vi "Zoom.vi"(2 "Final Zoom":sgl, 3 "Scene.Object IN":refnum<vi>) -> (1 "Scene.Object Out":refnum<vi>)   [LabVIEW 2010]
uses:
  <vilib>/Utility/miscctls.llb/LV3DPointTypeDef.ctl
  LVPresent_Globals.vi
  <vilib>/picture/3D Picture Control/NI_3D Picture Control.lvlib
panel:
  out "Transformation:Get Scale 2":T1
  out "Array":T1[](array[typedef])
  out "Transformation:Get Scale":T1
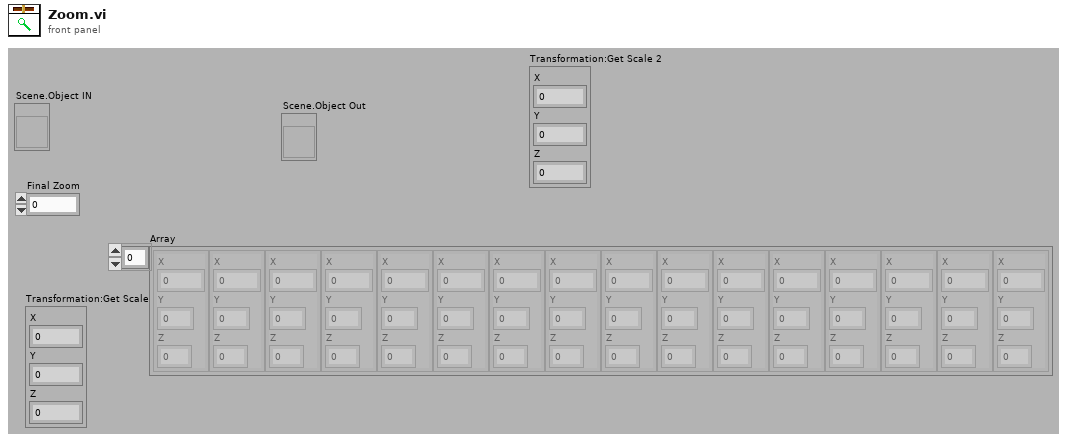
[diagram p1: front panel]
types:
  T1 = typedef "LV3DPointTypeDef.ctl" = cluster{"X":sgl, "Y":sgl, "Z":sgl}
  T2 = cluster{"Final Zoom":sgl, "Final Zoom":sgl, "Final Zoom":sgl}
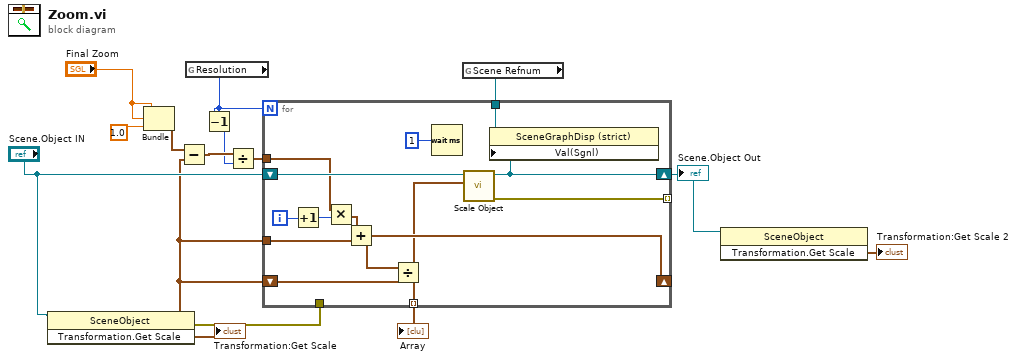
[diagram p0: block diagram]
diagram:
  n1 = invoke class="SceneObject" method="Transformation.Get Scale"(reference="Scene.Object IN") -> (error out=w6:errorcluster, "Transformation.Get Scale"=w8:T1)  [unwired: 2 in, 1 out]
  "Transformation:Get Scale" <- w8
  n2 = Bundle("Final Zoom"="Final Zoom", "Final Zoom"="Final Zoom", "Final Zoom"=sgl 1.0) -> (w13:T2)  [unwired: 1 in]
  n3 = Subtract(x=w13, y=w8) -> (x-y=w14:T1)
  n4 = global read "LVPresent_Globals.vi" "Resolution"() -> (w2:i32)
  n5 = Decrement(x=w2) -> (x-1=w1:i32)
  n6 = Divide(x=w14, y=w1) -> (x/y=w9:T1)
  n7 = global read "LVPresent_Globals.vi" "Scene Refnum"() -> (w3:refnum<vi>)
  n8 = for {
    N: w2 -> [_]
    shift-right: [w24] -> w5
    shift-left: "Scene.Object IN" -> [w20]
    tunnel: w8 -> [w25]
    tunnel: w3 -> [w23]
    shift-right: [w17] -> _
    shift-left: w8 -> [w18]
    tunnel: w9 -> [w19]
    tunnel: [w16] -> w7 mode=indexing
    tunnel: [w15] -> _ mode=indexing
    tunnel: w6 -> [_]
    i -> [w27]
    n9 = Increment(x=w27) -> (x+1=w26:i32)
    n10 = Multiply(x=w19, y=w26) -> (x*y=w21:T1)
    n11 = Add(x=w21, y=w25) -> (x+y=w17:T1)
    n12 = Divide(x=w17, y=w18) -> (x/y=w16:T1)
    n13 = Wait (ms)(milliseconds to wait=u32 1) -> ()  [unwired: 1 out]
    n14 = call <vilib>:"Scale Object.vi"("Scale"=w16, "Scene.Object In"=w20) -> ("error out"=w15:errorcluster, "Scene.Object Out"=w24:refnum<vi>)  [unwired: 8 in]
    n15 = property class="SceneGraphDisp (strict)"(reference=w23, "Val(Sgnl)"=w24) -> ()  [unwired: 1 in, 2 out]
  }
  "Scene.Object Out" <- w5
  "Array" <- w7
  n16 = invoke class="SceneObject" method="Transformation.Get Scale"(reference=w5) -> ("Transformation.Get Scale"=→"Transformation:Get Scale 2":T1)  [unwired: 2 in, 2 out]
